vi "Graph_Background_Size.vi"(0 "CenterPosX":dbl, 1 "XYGraph in":refnum<vi>, 5 "CenterPosY":dbl, 7 "Image Width":dbl=20.0, 9 "Image Height":dbl=20.0, 11 "error in (no error)":errorcluster, 12 "Bmp Path":string) -> (15 "error out":errorcluster)   [LabVIEW 2016]
uses:
  <vilib>/Utility/miscctls.llb/LVBoundsTypeDef.ctl
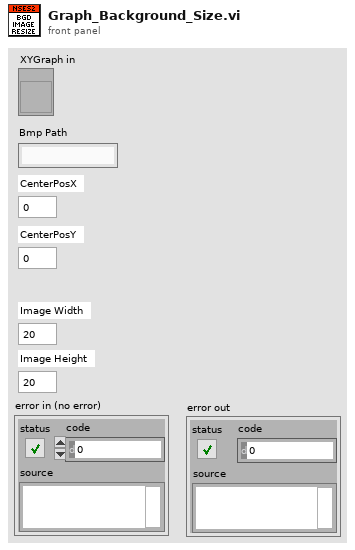
[diagram p1: front panel]
types:
  T1 = typedef "LVBoundsTypeDef.ctl" = cluster{"Width":u32, "Height":u32}
  T2 = typedef "imagedata.ctl" = cluster{"image type":i32, "image depth":i32, "image":u8[], "mask":u8[], "colors":u32[], "Rectangle":cluster{"left":i16, "top":i16, "right":i16, "bottom":i16}}
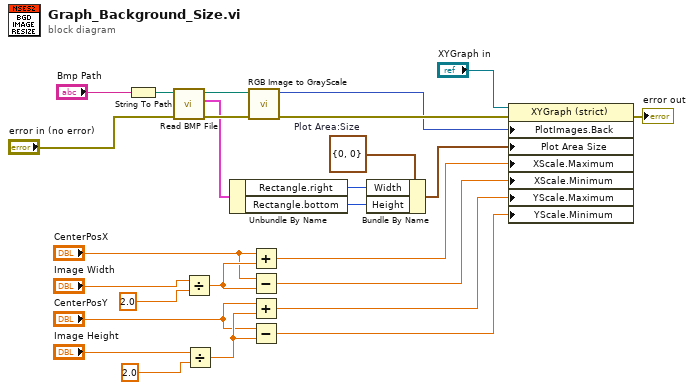
[diagram p0: block diagram]
diagram:
  w9 = T1 {"Width"=0, "Height"=0}  # Plot Area:Size
  n1 = String To Path(string="Bmp Path") -> (path=w24:path)
  n2 = call <vilib>:"Read BMP File.vi"("error in (no error)"="error in (no error)", "path to BMP file"=w24) -> ("error out"=w18:errorcluster, "image data"=w8:T2)  [unwired: 7 in, 1 out]
  n3 = Divide(x="Image Width", y=2.0) -> (x/y=w6:dbl)
  n4 = Divide(x="Image Height", y=2.0) -> (x/y=w21:dbl)
  n5 = Unbundle By Name(w8) -> ("Rectangle.right"=w16:i16, "Rectangle.bottom"=w17:i16)
  n6 = call "RGB Image to GrayScale.vi"("error in (no error)"=w18, "path to BMP file"=w24) -> ("error out"=w23:errorcluster, "RGB GrayScale"=w10:picture)  [unwired: 6 in]
  n7 = Add(x="CenterPosX", y=w6) -> (x+y=w12:dbl)
  n8 = Subtract(x="CenterPosX", y=w6) -> (x-y=w13:dbl)
  n9 = Add(x="CenterPosY", y=w21) -> (x+y=w14:dbl)
  n10 = Subtract(x="CenterPosY", y=w21) -> (x-y=w15:dbl)
  n11 = Bundle By Name(cluster=w9, "Width"=w16, "Height"=w17) -> (w11:T1)
  n12 = property on="Property Node" class="XYGraph (strict)"(reference="XYGraph in", error in=w23, "PlotImages.Back"=w10, "Plot Area Size"=w11, "XScale.Maximum"=w12, "XScale.Minimum"=w13, "YScale.Maximum"=w14, "YScale.Minimum"=w15) -> (error out=→"error out":errorcluster)  [unwired: 1 out]
